vi "init.vi"(8 "error in (no error)":errorcluster, 10 "Config Path":path, 11 "Dynamic-System in":refnum<class "Dynamic-System.lvclass">) -> (0 "error out":errorcluster, 3 "Dynamic-System out":refnum<class "Dynamic-System.lvclass">)   [LabVIEW 2025, in "Dynamic-System.lvclass"]
uses:
  Dynamic-System.lvclass
  Dynamic-System.lvclass/Dynamic-System.ctl
  d3891b41-4f08-416e-a85c-8f4602829767.vi
  <vilib>/JDP Science/JSONtext/JSON text to Variant.vi
  <vilib>/JDP Science/JSONtext/LVClass Serializer/JSONtext LVClass Serializer.lvclass
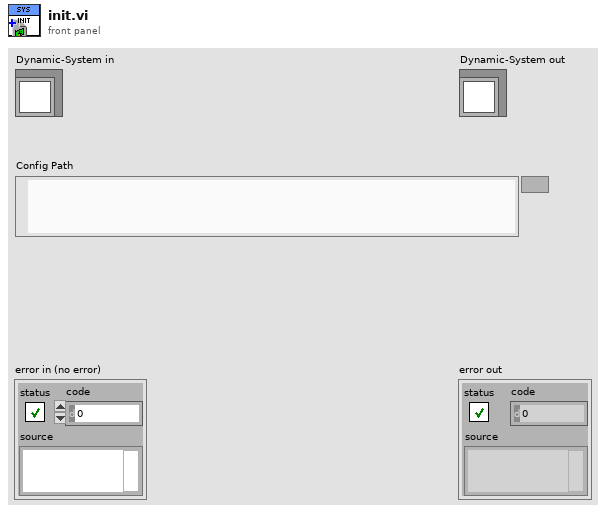
[diagram p1: front panel]
types:
  T1 = cluster{"State_Equations":string[], "State_Variables":string[], "Initial_Conditions":dbl[], "Step_size":dbl, "Data":dbl[][], "Parameters":cluster{"Param1":dbl, "Param2":dbl}}
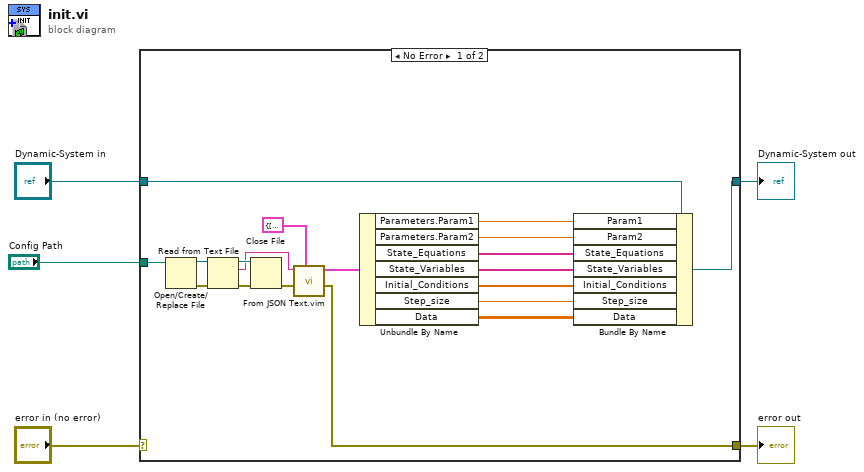
[diagram p0: block diagram]
diagram:
  n1 = case shown="No Error" "error in (no error)" {
    selector: "error in (no error)" -> [_ w26]
    tunnel: [w15 w26] -> w4
    tunnel: [w24 w25] -> w2
    tunnel: "Dynamic-System in" -> [w16 w25]
    tunnel: "Config Path" -> [w17 _]
    frame No Error {
      n2 = Open/Create/Replace File(file path (use dialog)=w17) -> (refnum out=w20:refnum<file>, error out=w23:errorcluster)  [unwired: 5 in, 1 out]
      n3 = Read from Text File(file (use dialog)=w20, error in=w23) -> (refnum out=w21:refnum<file>, text=w19:string, error out=w22:errorcluster)  [unwired: 2 in, 1 out]
      n4 = Close File(refnum=w21, error in=w22) -> (error out=w18:errorcluster)  [unwired: 1 out]
      n5 = call "From JSON Text.vim"("Data Type and Default Value"=T1 {"State_Equations"=[], "State_Variables"=[], "Initial_Conditions"=[], "Step_size"=0.0, "Data"=[], "Parameters"={"Param1"=0.0, "Param2"=0.0}}, "error in (no error)"=w18, "JSON"=w19) -> ("error out"=w15:errorcluster, "Data out"=w6:T1)  [unwired: 7 in]
      n6 = Unbundle By Name(w6) -> ("Parameters.Param1"=w12:dbl, "Parameters.Param2"=w11:dbl, "State_Equations"=w10:string[], "State_Variables"=w9:string[], "Initial_Conditions"=w13:dbl[], "Step_size"=w8:dbl, "Data"=w7:dbl[][])
      n7 = Bundle By Name(cluster=w16, "Param1"=w12, "Param2"=w11, "State_Equations"=w10, "State_Variables"=w9, "Initial_Conditions"=w13, "Step_size"=w8, "Data"=w7) -> (w24:refnum<class "Dynamic-System.lvclass">)
    }
    frame Error {
    }
  }
  "error out" <- w4
  "Dynamic-System out" <- w2
